vi "Get Sensor Attribute.vi"(8 "error in (no error)":errorcluster caption="错误输入（无错误）", 9 "value":u32, 10 "attribute":i32, 11 "sensorHandle":i32) -> (0 "error out":errorcluster caption="错误输出", 1 "value out":u32, 3 "function return":i32)   [LabVIEW 2018]
doc: "extern int __stdcall APSxGetSensorAttribute (int sensorHandle, IN int attribute, OUT void * value);"
uses:
  APSx.dll/APSx.dll
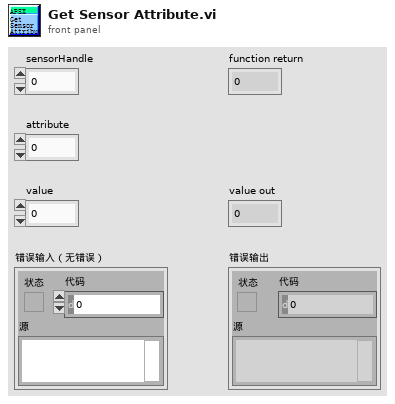
[diagram p1: front panel]
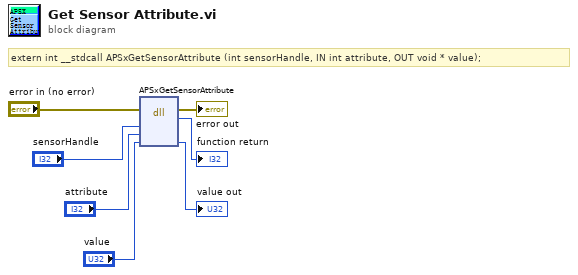
[diagram p0: block diagram]
diagram:
  # "extern int __stdcall APSxGetSensorAttribute (int sensorHandle, IN int attribute, OUT void * value);"
  n1 = dll-call lib="PTH2[abs D项目Feng恒隆项目Labview传感器对中台SourcesAPSx.dllAPSx.*" fn="APSxGetSensorAttribute"(error in="error in (no error)", "sensorHandle"="sensorHandle", "attribute"="attribute", "value"="value") -> (error out=→"error out":errorcluster, →"function return":i32, "value"=→"value out":u32)  [unwired: 4 in, 1 out]
